vi "TEB INIT.vi"   [LabVIEW 2019]
uses:
  e1039-target-controls/PDP/TPS Global.vi
  TEB Global.vi
  <vilib>/Utility/config.llb/NI_LVConfig.lvlib
types:
  T1 = typedef "NI_LVConfig.lvlib/Config Data RefNum.ctl" = refnum<k1>
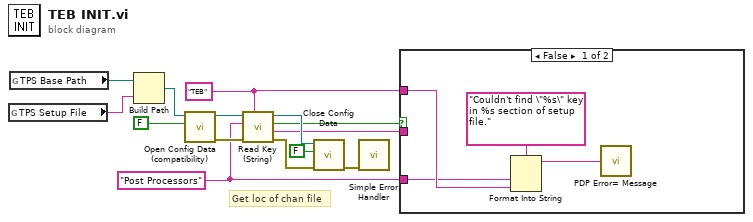
[diagram p0: block diagram]
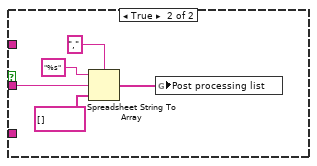
[diagram p2: hidden frame]
diagram:
  w4 = "TEB" ("section")
  w3 = "Post Processors" ("key")
  # "Get loc of chan file"
  n1 = global read "TPS Global.vi" "TPS Setup File"() -> (w7:string)
  n2 = global read "TPS Global.vi" "TPS Base Path"() -> (w14:path)
  n3 = Build Path(base path=w14, name or relative path=w7) -> (appended path=w8:path)
  n4 = call <vilib>:"Open Config Data (compatibility).vi"("create file if necessary (T)"=FALSE ("create file if necessary? (T)"), "configuration file path"=w8) -> ("error out"=w10:errorcluster, "refnum"=w11:T1)  [unwired: 7 in, 1 out]
  n5 = call <vilib>:"Read Key (String).vi"("section"=w4, "error in (no error)"=w10, "key"=w3, "refnum"=w11) -> ("error out"=w13:errorcluster, "value"=w6:string, "found?"=w5:bool, "refnum out"=w12:T1)  [unwired: 4 in]
  n6 = call <vilib>:"Close Config Data.vi"("error in (no error)"=w13, "write file if changed (T)"=FALSE, "refnum"=w12) -> ("error out"=w2:errorcluster)  [unwired: 7 in, 1 out]
  n7 = call <vilib>:"Simple Error Handler.vi"("error in (no error)"=w2) -> ()  [unwired: 4 in, 5 out]
  n8 = case shown="False" w5 {
    tunnel: w6 -> [_ w23]
    tunnel: w4 -> [w17 _]
    tunnel: w3 -> [w16 _]
    frame False {
      n9 = Format Into String(format string="Couldn't find \"%s\" key in %s section of setup file." ("Format String"), w16, w17) -> (resulting string=w15:string)  [unwired: 2 in, 1 out]
      n10 = call "PDP Error= Message.vi"("Message"=w15) -> ()
    }
    frame True {
      n11 = Spreadsheet String To Array(delimiter (Tab)=",", format string="%s", spreadsheet string=w23, array type (2D Dbl)=string[] [] ("Array Constant")) -> (array=w19:string[])
      n12 = global write "TEB Global.vi" "Post processing list"(w19) -> ()
    }
  }
